vi "Leader8.vi"   [LabVIEW 2016]
uses:
  <vilib>/NXT/Block Support/NXT_TimerIndex.ctl
  <vilib>/NXT/Block Support/NXT_OutputPort.ctl
  <vilib>/NXT/Block Support/NXT_InputPort.ctl
  <vilib>/NXT/Dual Mode Library/Motors/ResetMotor.vi
  <vilib>/NXT/Dual Mode Library/Sensors/Reset_Timer.vi
  <vilib>/NXT/Dual Mode Library/Sensors/EV3_Color_Reflect.vi
  <vilib>/NXT/Dual Mode Library/Sensors/EV3_Gyro_Angle.vi
  <vilib>/NXT/Dual Mode Library/Sensors/Touch_Pressed.vi
  <vilib>/NXT/Dual Mode Library/Display/drawText.vi
  <vilib>/NXT/Dual Mode Library/Sensors/Read_Timer.vi
  <vilib>/NXT/Dual Mode Library/Display/drawNumber.vi
  <vilib>/NXT/Dual Mode Library/Motors/Rotation.vi
  <vilib>/NXT/Dual Mode Library/Sensors/EV3_Gyro_Reset.vi
  <vilib>/NXT/Dual Mode Library/Sensors/EV3_Gyro_Rate.vi
  <vilib>/NXT/Dual Mode Library/Display/drawNumber_float.vi
  <vilib>/NXT/Dual Mode Library/prims/inRangeAndCoerce/inRangeAndCoerce_float.vi
  <vilib>/NXT/NXTIO Xnodes/NXTIONodeSubVIs/NXTMoveMotors.vi
  <vilib>/NXT/Dual Mode Library/Display/drawText_Right.vi
  <vilib>/NXT/NXTIO Xnodes/NXTIONodeSubVIs/NXTStopMotors.vi
  <vilib>/NXT/Subs/LVHSConnector.ctl
  <vilib>/NXT/NXTIO Xnodes/AddressXNode/NXTIOAddress.xnode
  <vilib>/NXT/NXTIO Xnodes/NXTIOXNode/NXTIO.xnode
  <vilib>/NXT/LegoClasses/BrickReference/BrickReference.lvclass
types:
  T1 = typedef "LVHSConnector.ctl" = refnum<class "BrickReference.lvclass">
  T2 = typedef "NXT_InputPort.ctl" = u32
  T3 = typedef "NXT_OutputPort.ctl" = u8
  T4 = typedef "NXT_TimerIndex.ctl" = u8
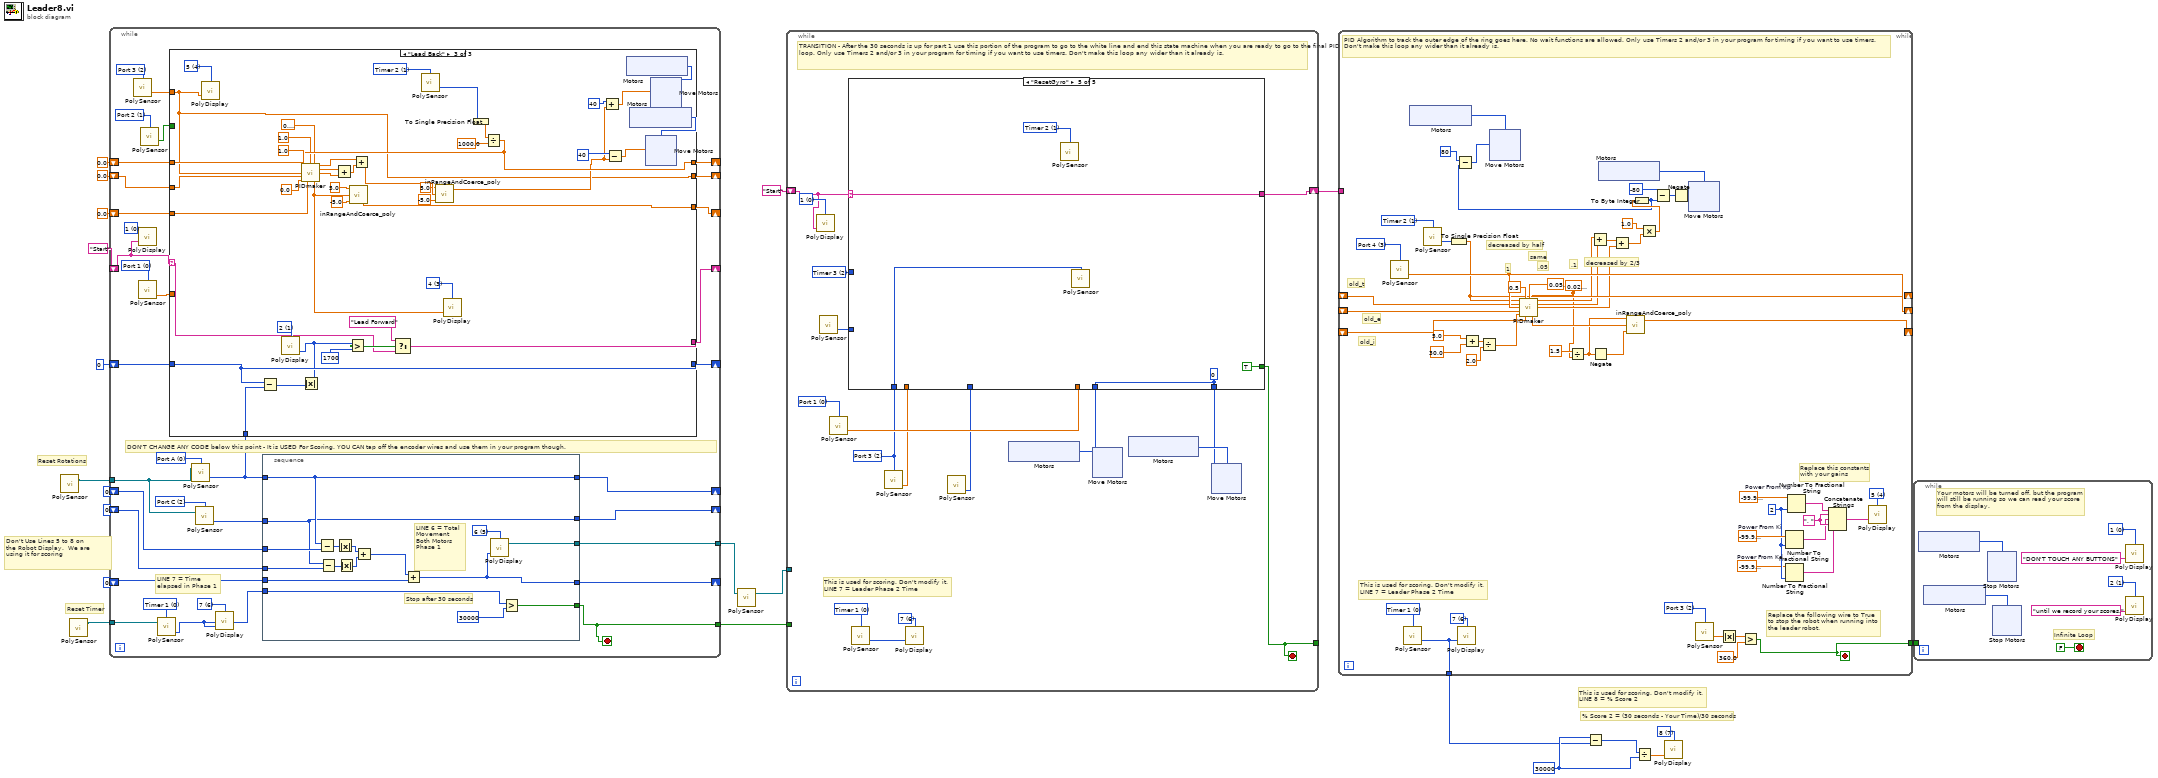
[diagram p0: block diagram]
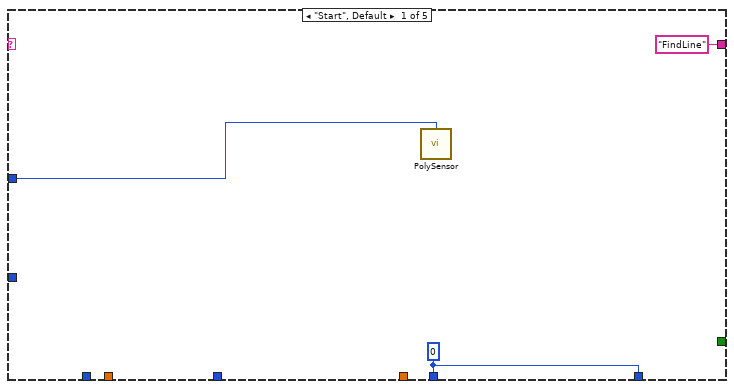
[diagram p2: hidden frame]
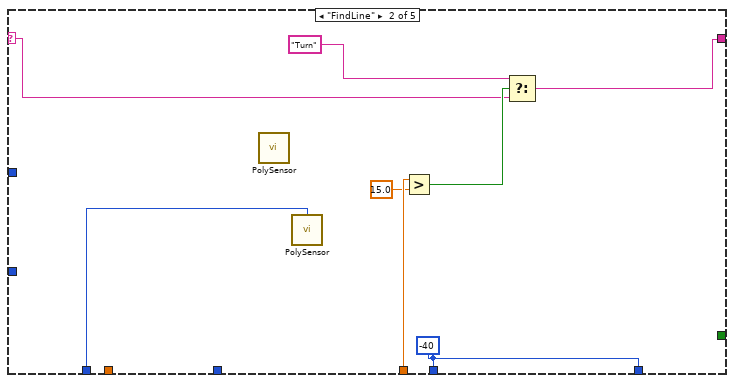
[diagram p3: hidden frame]
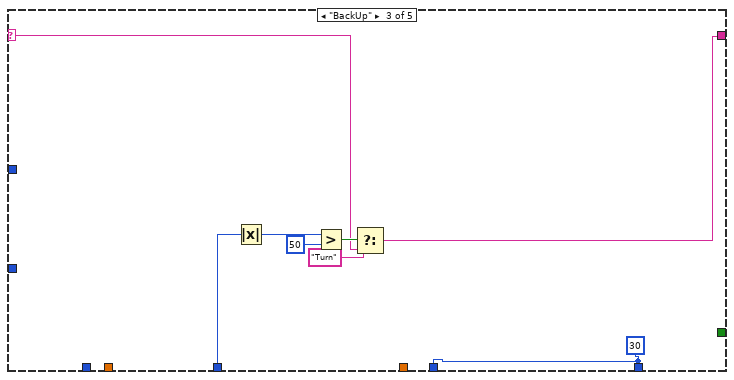
[diagram p4: hidden frame]
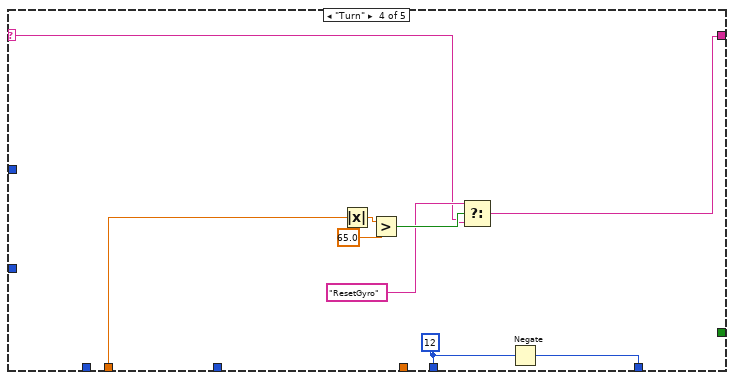
[diagram p5: hidden frame]
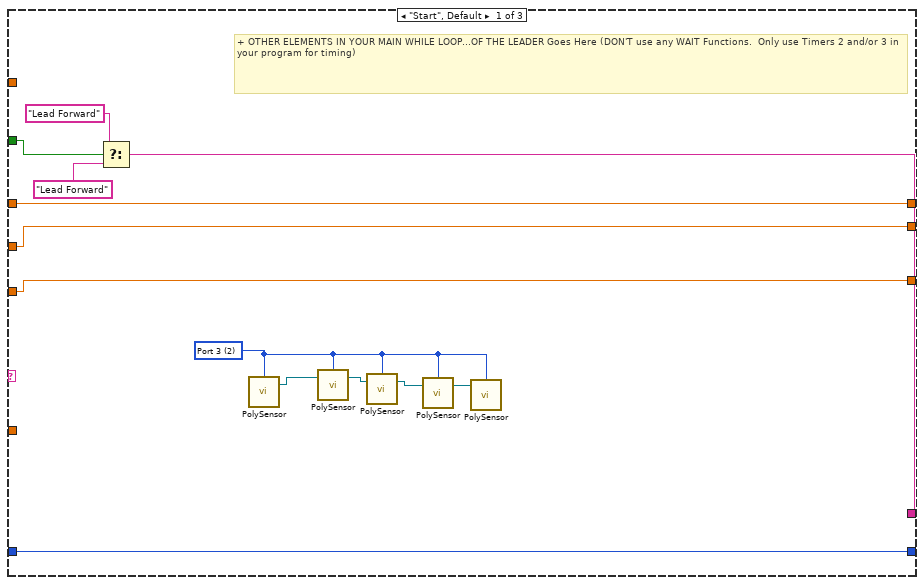
[diagram p6: hidden frame]
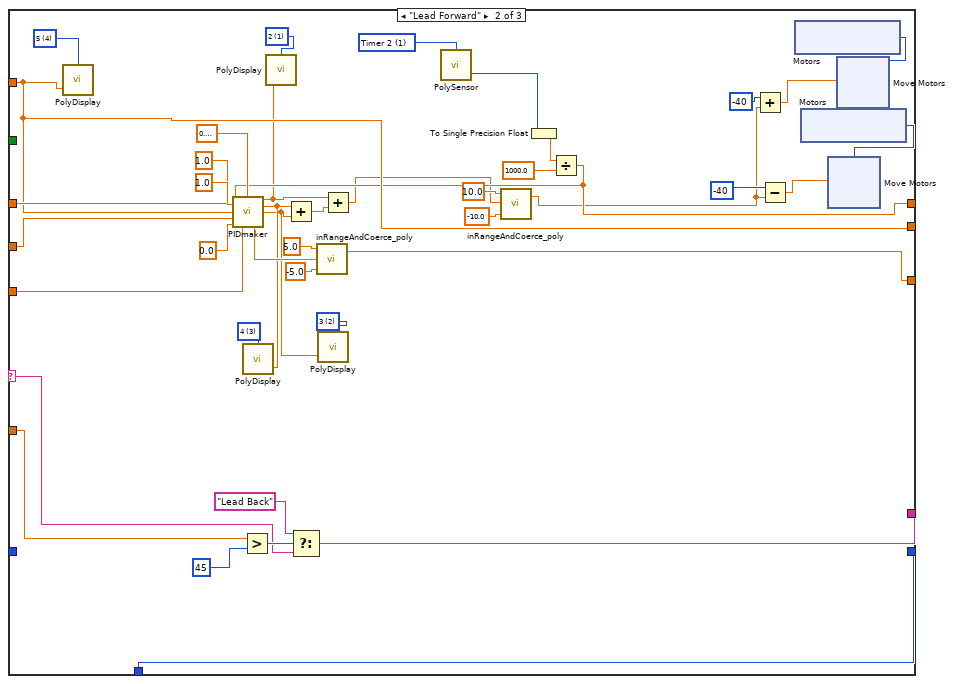
[diagram p7: hidden frame]
diagram:
  w6 = u32 30000 ("Value (msec)")
  w7 = i16 7 items=["1", "2", "3", "4", "5", "6", "7", "8", "9", "10", "11", "12"] ("Line")
  # "This is used for scoring. Don't modify it.\nLINE 8 = % Score 2"
  # "% Score 2 = (30 seconds - Your Time)/30 seconds"
  # "Don't Use Lines 5 to 8 on\nthe Robot Display.  We are \nusing it for scoring"
  # "Reset Timer"
  # "Reset Rotations"
  n1 = call-poly <vilib>:"PolySensor.vi"() -> ("NXT/EV3"=w18:T1)  [unwired: 4 in]
  n2 = call-poly <vilib>:"PolySensor.vi"() -> ("NXT/EV3"=w17:T1)  [unwired: 4 in]
  n3 = while {
    tunnel: w18 -> [w55]
    shift-right: [w50] -> _
    shift-left: 0 ("Angle of Rotation") -> [w52]
    shift-right: [w49] -> _
    shift-left: 0 ("Angle of Rotation") -> [w51]
    shift-right: [w53] -> _
    shift-left: 0 -> [w54]
    tunnel: w17 -> [w47]
    tunnel: [w24] -> w1
    tunnel: [w42] -> w16
    shift-right: [w36] -> _
    shift-left: 0 -> [w37]
    shift-right: [w32] -> _
    shift-left: "Start" -> [w31]
    shift-right: [w26] -> _
    shift-left: sgl 0.0 -> [w29]
    shift-right: [w25] -> _
    shift-left: sgl 0.0 ("Degrees") -> [w30]
    shift-right: [w27] -> _
    shift-left: sgl 0.0 ("coerced(x)") -> [w28]
    stop <- w24 stop-if-true
    w23 = T2 1 items=["Port 1", "Port 2", "Port 3", "Port 4"] ("Port (Port 1)")
    w33 = i16 0 items=["1", "2", "3", "4", "5", "6", "7", "8", "9", "10", "11", "12"] ("Line")
    w35 = T2 2 items=["Port 1", "Port 2", "Port 3", "Port 4"] ("Port (Port 1)")
    w38 = T2 0 items=["Port 1", "Port 2", "Port 3", "Port 4"] ("Port (Port 1)")
    w44 = i16 6 items=["1", "2", "3", "4", "5", "6", "7", "8", "9", "10", "11", "12"] ("Line")
    w45 = T3 0 items=["Port A", "Port B", "Port C", "Port D"] ("Port (Port A)")
    w46 = T3 2 items=["Port A", "Port B", "Port C", "Port D"] ("Port (Port A)")
    w48 = T4 0 items=["Timer 1", "Timer 2", "Timer 3"] ("Timer (Timer 1)")
    # "DON'T CHANGE ANY CODE below this point - It is USED For Scoring. YOU CAN tap off the encoder wires and use them in your program though."
    # "LINE 7 = Time elapsed in Phase 1"
    n4 = call-poly <vilib>:"PolySensor.vi"("Port (Port 1)"=w35) -> ("Degrees"=w34:sgl)  [unwired: 2 in, 1 out]
    n5 = call-poly <vilib>:"PolyDisplay.vi"("Text"=w31, "Line"=w33) -> ()  [unwired: 2 in, 1 out]
    n6 = call-poly <vilib>:"PolySensor.vi"("Port (Port 1)"=w38) -> ("Scaled Value"=w22:sgl)  [unwired: 2 in, 1 out]
    n7 = call-poly <vilib>:"PolySensor.vi"("Port (Port 1)"=w23) -> ("Yes / No"=w41:bool)  [unwired: 2 in, 1 out]
    n8 = call-poly <vilib>:"PolySensor.vi"("NXT/EV3"=w47, "Timer (Timer 1)"=w48) -> ("Value (msec)"=w43:u32)  [unwired: 1 in, 1 out]
    n9 = call-poly <vilib>:"PolySensor.vi"("NXT/EV3"=w55, "Port (Port A)"=w45) -> ("Angle of Rotation"=w40:i32)  [unwired: 1 in, 1 out]
    n10 = case shown="\"Lead Back\"" w31 {
      selector: w31 -> [_ w106 w160]
      tunnel: [w67 w107 w164] -> w32
      tunnel: w41 -> [w68 _ _]
      tunnel: w40 -> [_ w104 w161]
      tunnel: w37 -> [w65 _ w159]
      tunnel: w22 -> [_ w105 _]
      tunnel: [w65 w104 w159] -> w36
      tunnel: w34 -> [_ w81 w127]
      tunnel: w30 -> [w63 w86 w145]
      tunnel: w29 -> [w64 w87 w144]
      tunnel: w28 -> [w62 w85 w139]
      tunnel: [w62 w84 w138] -> w27
      tunnel: [w64 w80 w135] -> w26
      tunnel: [w63 w81 w127] -> w25
      frame "Start", Default {
        w57 = T2 2 items=["Port 1", "Port 2", "Port 3", "Port 4"] ("Port (Port 1)")
        # "+ OTHER ELEMENTS IN YOUR MAIN WHILE LOOP...OF THE LEADER Goes Here (DON'T use any WAIT Functions.  Only use Timers 2 and/or 3 in your program for timing)"
        n11 = Select(t="Lead Forward", s=w68, f="Lead Forward") -> (s? t:f=w67:string)
        n12 = call-poly <vilib>:"PolySensor.vi"("Port (Port 1)"=w57) -> ("NXT/EV3"=w58:T1)  [unwired: 3 in]
        n13 = call-poly <vilib>:"PolySensor.vi"("NXT/EV3"=w58, "Port (Port 1)"=w57) -> ("NXT/EV3"=w59:T1)  [unwired: 1 in, 1 out]
        n14 = call-poly <vilib>:"PolySensor.vi"("NXT/EV3"=w59, "Port (Port 1)"=w57) -> ("NXT/EV3"=w61:T1)  [unwired: 1 in, 1 out]
        n15 = call-poly <vilib>:"PolySensor.vi"("NXT/EV3"=w61, "Port (Port 1)"=w57) -> ("NXT/EV3"=w60:T1)  [unwired: 1 in, 1 out]
        n16 = call-poly <vilib>:"PolySensor.vi"("NXT/EV3"=w60, "Port (Port 1)"=w57) -> ()  [unwired: 2 in, 1 out]
      }
      frame "Lead Forward" {
        w70 = i16 2 items=["1", "2", "3", "4", "5", "6", "7", "8", "9", "10", "11", "12"] ("Line")
        w72 = i16 1 items=["1", "2", "3", "4", "5", "6", "7", "8", "9", "10", "11", "12"] ("Line")
        w75 = i16 3 items=["1", "2", "3", "4", "5", "6", "7", "8", "9", "10", "11", "12"] ("Line")
        w82 = i16 4 items=["1", "2", "3", "4", "5", "6", "7", "8", "9", "10", "11", "12"] ("Line")
        w92 = T4 1 items=["Timer 1", "Timer 2", "Timer 3"] ("Timer (Timer 1)")
        n17 = call-poly <vilib>:"PolyDisplay.vi"("number"=w81, "Line"=w82) -> ()  [unwired: 2 in, 1 out]
        n18 = Greater?(x=w105, y=45) -> (0:w108:bool)
        n19 = Select(t="Lead Back", s=w108, f=w106) -> (s? t:f=w107:string)
        n20 = call-poly <vilib>:"PolySensor.vi"("Timer (Timer 1)"=w92) -> ("Value (msec)"=w91:u32)  [unwired: 2 in, 1 out]
        n21 = To Single Precision Float(number=w91) -> (single precision float=w89:sgl)
        n22 = Divide(x=w89, y=sgl 1000.0) -> (x/y=w80:sgl)
        n23 = call "PIDmaker.vi"("New Time"=w80, "Kp"=sgl 1.0, "Kd"=sgl 1.0, "Ki"=sgl 0.1, "Old Time"=w87, "New Value"=w81, "Old Value"=w86, "Desired Value"=sgl 0.0, "Integral In"=w85) -> ("P out"=w73:sgl, "D out"=w71:sgl, "I out"=w69:sgl, "Integral Out"=w74:sgl)  [unwired: 3 in]
        n24 = call-poly <vilib>:"PolyDisplay.vi"("number"=w71, "Line"=w75) -> ()  [unwired: 2 in, 1 out]
        n25 = call-poly <vilib>:"PolyDisplay.vi"("number"=w73, "Line"=w72) -> ()  [unwired: 2 in, 1 out]
        n26 = Add(x=w71, y=w69) -> (x+y=w100:sgl)
        n27 = call-poly <vilib>:"inRangeAndCoerce_poly.vi"("lower limit"=sgl -5.0, "x"=w74, "upper limit"=sgl 5.0) -> ("coerced(x)"=w84:sgl)  [unwired: 1 out]
        n28 = call-poly <vilib>:"PolyDisplay.vi"("number"=w69, "Line"=w70) -> ()  [unwired: 2 in, 1 out]
        n29 = Add(x=w73, y=w100) -> (x+y=w77:sgl)
        n30 = call-poly <vilib>:"inRangeAndCoerce_poly.vi"("lower limit"=sgl -10.0, "x"=w77, "upper limit"=sgl 10.0) -> ("coerced(x)"=w76:sgl)  [unwired: 1 out]
        n31 = Add(x=-40, y=w76) -> (x+y=w93:sgl)
        n32 = Subtract(x=-40, y=w76) -> (x-y=w83:sgl)
        n33 = xnode "Motors"() -> ("Motor"=w103:T3)
        n34 = xnode "Motors"() -> ("Motor"=w88:T3)
        n35 = xnode "Move Motors"("Power/Speed 1"=w83, "Motors"=w88) -> ()  [unwired: 1 in, 1 out]
        n36 = xnode "Move Motors"("Power/Speed 1"=w93, "Motors"=w103) -> ()  [unwired: 1 in, 1 out]
      }
      frame "Lead Back" {
        w128 = i16 4 items=["1", "2", "3", "4", "5", "6", "7", "8", "9", "10", "11", "12"] ("Line")
        w143 = T4 1 items=["Timer 1", "Timer 2", "Timer 3"] ("Timer (Timer 1)")
        w165 = i16 3 items=["1", "2", "3", "4", "5", "6", "7", "8", "9", "10", "11", "12"] ("Line")
        w168 = i16 1 items=["1", "2", "3", "4", "5", "6", "7", "8", "9", "10", "11", "12"] ("Line")
        n37 = call-poly <vilib>:"PolyDisplay.vi"("number"=w127, "Line"=w128) -> ()  [unwired: 2 in, 1 out]
        n38 = Subtract(x=w159, y=w161) -> (x-y=w158:i32)
        n39 = Absolute Value(x=w158) -> (abs(x)=w157:i32)
        n40 = call-poly <vilib>:"PolyDisplay.vi"("number"=w157, "Line"=w168) -> ()  [unwired: 2 in, 1 out]
        n41 = Greater?(x=w157, y=1700) -> (0:w162:bool)
        n42 = Select(t="Lead Forward", s=w162, f=w160) -> (s? t:f=w164:string)
        n43 = call-poly <vilib>:"PolySensor.vi"("Timer (Timer 1)"=w143) -> ("Value (msec)"=w142:u32)  [unwired: 2 in, 1 out]
        n44 = To Single Precision Float(number=w142) -> (single precision float=w140:sgl)
        n45 = Divide(x=w140, y=sgl 1000.0) -> (x/y=w135:sgl)
        n46 = call "PIDmaker.vi"("New Time"=w135, "Kp"=sgl 1.0, "Kd"=sgl 1.0, "Ki"=sgl 0.1, "Old Time"=w144, "New Value"=w127, "Old Value"=w145, "Desired Value"=sgl 0.0, "Integral In"=w139) -> ("P out"=w152:sgl, "D out"=w153:sgl, "I out"=w150:sgl, "Integral Out"=w137:sgl)  [unwired: 3 in]
        n47 = Add(x=w153, y=w150) -> (x+y=w154:sgl)
        n48 = call-poly <vilib>:"inRangeAndCoerce_poly.vi"("lower limit"=sgl -5.0, "x"=w137, "upper limit"=sgl 5.0) -> ("coerced(x)"=w138:sgl)  [unwired: 1 out]
        n49 = Add(x=w152, y=w154) -> (x+y=w132:sgl)
        n50 = call-poly <vilib>:"inRangeAndCoerce_poly.vi"("lower limit"=sgl -5.0, "x"=w132, "upper limit"=sgl 5.0) -> ("coerced(x)"=w131:sgl)  [unwired: 1 out]
        n51 = call-poly <vilib>:"PolyDisplay.vi"("number"=w137, "Line"=w165) -> ()  [unwired: 2 in, 1 out]
        n52 = Add(x=40, y=w131) -> (x+y=w146:sgl)
        n53 = Subtract(x=40, y=w131) -> (x-y=w136:sgl)
        n54 = xnode "Motors"() -> ("Motor"=w166:T3)
        n55 = xnode "Motors"() -> ("Motor"=w167:T3)
        n56 = xnode "Move Motors"("Power/Speed 1"=w136, "Motors"=w167) -> ()  [unwired: 1 in, 1 out]
        n57 = xnode "Move Motors"("Power/Speed 1"=w146, "Motors"=w166) -> ()  [unwired: 1 in, 1 out]
      }
    }
    n58 = call-poly <vilib>:"PolySensor.vi"("NXT/EV3"=w55, "Port (Port A)"=w46) -> ("Angle of Rotation"=w39:i32)  [unwired: 1 in, 1 out]
    n59 = call-poly <vilib>:"PolyDisplay.vi"("number"=w43, "Line"=w44) -> ()  [unwired: 2 in, 1 out]
    n60 = stacked-sequence {
      tunnel: w54 -> [w201]
      tunnel: [w188] -> w53
      tunnel: w43 -> [w199]
      tunnel: [w198] -> w24
      tunnel: w40 -> [w191]
      tunnel: w39 -> [w190]
      tunnel: w52 -> [w193]
      tunnel: w51 -> [w192]
      tunnel: [w191] -> w50
      tunnel: [w190] -> w49
      tunnel: [w186] -> w42
      frame #0 {
        w187 = i16 5 items=["1", "2", "3", "4", "5", "6", "7", "8", "9", "10", "11", "12"] ("Line")
        # "LINE 6 = Total\nMovement\nBoth Motors\nPhase 1"
        # "Stop after 30 seconds"
        n61 = Subtract(x=w191, y=w193) -> (x-y=w197:i32)
        n62 = Subtract(x=w190, y=w192) -> (x-y=w196:i32)
        n63 = Absolute Value(x=w197) -> (abs(x)=w195:i32)
        n64 = Absolute Value(x=w196) -> (abs(x)=w194:i32)
        n65 = Add(x=w195, y=w194) -> (x+y=w189:i32)
        n66 = Add(x=w189, y=w201) -> (x+y=w188:i32)
        n67 = call-poly <vilib>:"PolyDisplay.vi"("number"=w188, "Line"=w187) -> ("NXT/EV3"=w186:T1)  [unwired: 2 in]
        n68 = Greater?(x=w199, y=u32 30000 ("Value (msec)")) -> (0:w198:bool)
      }
    }
  }
  n69 = call-poly <vilib>:"PolySensor.vi"("NXT/EV3"=w16) -> ("NXT/EV3"=w2:T1)  [unwired: 3 in]
  n70 = while {
    shift-right: [w206] -> w8
    shift-left: "Start" -> [w202]
    tunnel: [w204] -> _
    tunnel: w2 -> [_]
    tunnel: w1 -> [_]
    stop <- w204 stop-if-true
    w203 = i16 0 items=["1", "2", "3", "4", "5", "6", "7", "8", "9", "10", "11", "12"] ("Line")
    w205 = T2 0 items=["Port 1", "Port 2", "Port 3", "Port 4"] ("Port (Port 1)")
    w209 = T2 2 items=["Port 1", "Port 2", "Port 3", "Port 4"] ("Port (Port 1)")
    w214 = T4 2 items=["Timer 1", "Timer 2", "Timer 3"] ("Timer (Timer 1)")
    w217 = i16 6 items=["1", "2", "3", "4", "5", "6", "7", "8", "9", "10", "11", "12"] ("Line")
    w219 = T4 0 items=["Timer 1", "Timer 2", "Timer 3"] ("Timer (Timer 1)")
    # "This is used for scoring. Don't modify it.\nLINE 7 = Leader Phase 2 Time"
    # "TRANSITION - After the 30 seconds is up for part 1 use this portion of the program to go to the white line and end this state machine when you are ready to go to the final PID control loop. Only use Timers 2 and/or 3 in your program for timing if you want to use timers. Don't make this loop any wider than it already is."
    n71 = call-poly <vilib>:"PolyDisplay.vi"("Text"=w202, "Line"=w203) -> ()  [unwired: 2 in, 1 out]
    n72 = call-poly <vilib>:"PolySensor.vi"() -> ("Value (msec)"=w213:u32)  [unwired: 3 in, 1 out]
    n73 = call-poly <vilib>:"PolySensor.vi"("Port (Port 1)"=w205) -> ("Scaled Value"=w210:sgl)  [unwired: 2 in, 1 out]
    n74 = call-poly <vilib>:"PolySensor.vi"("Timer (Timer 1)"=w219) -> ("Value (msec)"=w218:u32)  [unwired: 2 in, 1 out]
    n75 = call-poly <vilib>:"PolySensor.vi"("Port (Port 1)"=w209) -> ("Degrees"=w208:sgl)  [unwired: 2 in, 1 out]
    n76 = call-poly <vilib>:"PolyDisplay.vi"("number"=w218, "Line"=w217) -> ()  [unwired: 2 in, 1 out]
    n77 = call-poly <vilib>:"PolySensor.vi"() -> ("Angle of Rotation"=w207:i32)  [unwired: 3 in, 1 out]
    n78 = case shown="\"ResetGyro\"" w202 {
      selector: w202 -> [_ w241 w249 w256 w266]
      tunnel: ["FindLine" w243 w247 w255 w266] -> w206
      tunnel: w214 -> [w238 _ _ _ _]
      tunnel: w213 -> [_ _ _ _ _]
      tunnel: [w236 w239 w254 w263 w265] -> w212
      tunnel: [w236 w239 w254 w262 w265] -> w211
      tunnel: w210 -> [_ w246 _ _ _]
      tunnel: w209 -> [_ w240 _ _ w268]
      tunnel: w208 -> [_ _ _ w261 _]
      tunnel: w207 -> [_ _ w253 _ _]
      tunnel: [_ _ _ _ TRUE] -> w204
      frame "Start", Default {
        w236 = 0
        n79 = call-poly <vilib>:"PolySensor.vi"("Timer (Timer 1)"=w238) -> ()  [unwired: 3 in, 1 out]
      }
      frame "FindLine" {
        w239 = -40
        n80 = call-poly <vilib>:"PolySensor.vi"() -> ()  [unwired: 4 in, 1 out]
        n81 = call-poly <vilib>:"PolySensor.vi"("Port (Port 1)"=w240) -> ()  [unwired: 3 in, 1 out]
        n82 = Greater?(x=w246, y=sgl 15.0) -> (0:w244:bool)
        n83 = Select(t="Turn", s=w244, f=w241) -> (s? t:f=w243:string)
      }
      frame "BackUp" {
        w254 = 30
        n84 = Absolute Value(x=w253) -> (abs(x)=w251:i32)
        n85 = Greater?(x=w251, y=50) -> (0:w250:bool)
        n86 = Select(t="Turn", s=w250, f=w249) -> (s? t:f=w247:string)
      }
      frame "Turn" {
        w263 = 12
        n87 = Absolute Value(x=w261) -> (abs(x)=w260:sgl)
        n88 = Greater?(x=w260, y=sgl 65.0) -> (0:w258:bool)
        n89 = Select(t="ResetGyro", s=w258, f=w256) -> (s? t:f=w255:string)
        n90 = Negate(x=w263) -> (-x=w262:i32)
      }
      frame "ResetGyro" {
        w264 = T4 1 items=["Timer 1", "Timer 2", "Timer 3"] ("Timer (Timer 1)")
        w265 = 0
        n91 = call-poly <vilib>:"PolySensor.vi"("Timer (Timer 1)"=w264) -> ()  [unwired: 3 in, 1 out]
        n92 = call-poly <vilib>:"PolySensor.vi"("Port (Port 1)"=w268) -> ()  [unwired: 3 in, 1 out]
      }
    }
    n93 = xnode "Motors"() -> ("Motor"=w216:T3)
    n94 = xnode "Move Motors"("Power/Speed 1"=w212, "Motors"=w216) -> ()  [unwired: 1 in, 1 out]
    n95 = xnode "Motors"() -> ("Motor"=w215:T3)
    n96 = xnode "Move Motors"("Power/Speed 1"=w211, "Motors"=w215) -> ()  [unwired: 1 in, 1 out]
  }
  n97 = while {
    tunnel: [w273] -> w9
    tunnel: w8 -> [_]
    tunnel: [w320] -> w5
    shift-right: [w305] -> _
    shift-left: _ -> [w304]
    shift-right: [w301] -> _
    shift-left: _ -> [w300]
    shift-right: [w288] -> _
    shift-left: _ -> [w289]
    stop <- w273 stop-if-true
    w277 = T2 2 items=["Port 1", "Port 2", "Port 3", "Port 4"] ("Port (Port 1)")
    w286 = sgl 0.03 ("Ki")
    w307 = T4 1 items=["Timer 1", "Timer 2", "Timer 3"] ("Timer (Timer 1)")
    w308 = T2 3 items=["Port 1", "Port 2", "Port 3", "Port 4"] ("Port (Port 1)")
    w313 = ", " ("string")
    w316 = i16 2 ("precision (6)")
    w315 = sgl -99.9  # Power From Kd
    w317 = sgl -99.9  # Power From Ki
    w318 = sgl -99.9  # Power From Kp
    w319 = i16 4 items=["1", "2", "3", "4", "5", "6", "7", "8", "9", "10", "11", "12"] ("Line")
    w321 = i16 6 items=["1", "2", "3", "4", "5", "6", "7", "8", "9", "10", "11", "12"] ("Line")
    w322 = T4 0 items=["Timer 1", "Timer 2", "Timer 3"] ("Timer (Timer 1)")
    # "decreased by 2/3"
    # "same"
    # "decreased by half"
    # ".1"
    # ".05"
    # "1"
    # "old_i"
    # "old_e"
    # "old_t"
    # "Replace this constants\nwith your gains"
    # "This is used for scoring. Don't modify it.\nLINE 7 = Leader Phase 2 Time"
    # "PID Algorithm to track the outer edge of the ring goes here. No wait functions are allowed. Only use Timers 2 and/or 3 in your program for timing if you want to use timers.\nDon't make this loop any wider than it already is."
    # "Replace the following wire to True\nto stop the robot when running into \nthe leader robot."
    n98 = call-poly <vilib>:"PolySensor.vi"("Port (Port 1)"=w308) -> ("Scaled Value"=w305:sgl)  [unwired: 2 in, 1 out]
    n99 = call-poly <vilib>:"PolySensor.vi"("Timer (Timer 1)"=w322) -> ("Value (msec)"=w320:u32)  [unwired: 2 in, 1 out]
    n100 = xnode "Motors"() -> ("Motor"=w283:T3)
    n101 = call-poly <vilib>:"PolySensor.vi"("Timer (Timer 1)"=w307) -> ("Value (msec)"=w306:u32)  [unwired: 2 in, 1 out]
    n102 = To Single Precision Float(number=w306) -> (single precision float=w301:sgl)
    n103 = call-poly <vilib>:"PolyDisplay.vi"("number"=w320, "Line"=w321) -> ()  [unwired: 2 in, 1 out]
    n104 = Add(x=sgl 5.0, y=sgl 30.0) -> (x+y=w299:sgl)
    n105 = Divide(x=w299, y=sgl 2.0) -> (x/y=w296:sgl)
    n106 = call "PIDmaker.vi"("New Time"=w301, "Kp"=sgl 0.5, "Kd"=sgl 0.05, "Ki"=w286, "Old Time"=w300, "New Value"=w305, "Old Value"=w304, "Desired Value"=w296, "Integral In"=w289) -> ("P out"=w292:sgl, "D out"=w291:sgl, "I out"=w290:sgl, "Integral Out"=w295:sgl)  [unwired: 3 in]
    n107 = Divide(x=sgl 1.5, y=w286) -> (x/y=w284:sgl)
    n108 = Add(x=w292, y=w291) -> (x+y=w293:sgl)
    n109 = Negate(x=w284) -> (-x=w285:sgl)
    n110 = xnode "Motors"() -> ("Motor"=w309:T3)
    n111 = Add(x=w293, y=w290) -> (x+y=w279:sgl)
    n112 = call-poly <vilib>:"inRangeAndCoerce_poly.vi"("lower limit"=w285, "x"=w295, "upper limit"=w284) -> ("coerced(x)"=w288:sgl)  [unwired: 1 out]
    n113 = Multiply(x=sgl 1.0 ("Ki"), y=w279) -> (x*y=w271:sgl)
    n114 = To Byte Integer(number=w271) -> (8bit integer=w269:i8)
    n115 = Subtract(x=i8 80 ("Power/Speed 1"), y=w269) -> (x-y=w270:i8)
    n116 = xnode "Move Motors"("Power/Speed 1"=w270, "Motors"=w283) -> ()  [unwired: 1 in, 1 out]
    n117 = Subtract(x=i8 -80, y=w269) -> (x-y=w281:i8)
    n118 = Negate(x=w281) -> (-x=w280:i8)
    n119 = xnode "Move Motors"("Power/Speed 1"=w280, "Motors"=w309) -> ()  [unwired: 1 in, 1 out]
    n120 = call-poly <vilib>:"PolySensor.vi"("Port (Port 1)"=w277) -> ("Degrees"=w276:sgl)  [unwired: 2 in, 1 out]
    n121 = Absolute Value(x=w276) -> (abs(x)=w274:sgl)
    n122 = Greater?(x=w274, y=sgl 360.0) -> (0:w273:bool)
    n123 = Number To Fractional String(number=w317, precision (6)=w316) -> (F-format string=w312:string)  [unwired: 2 in]
    n124 = Number To Fractional String(number=w315, precision (6)=w316) -> (F-format string=w311:string)  [unwired: 2 in]
    n125 = Number To Fractional String(number=w318, precision (6)=w316) -> (F-format string=w314:string)  [unwired: 2 in]
    n126 = Concatenate Strings(w314, w313, w312, w313, w311) -> (w310:string)
    n127 = call-poly <vilib>:"PolyDisplay.vi"("Text"=w310, "Line"=w319) -> ()  [unwired: 2 in, 1 out]
  }
  n128 = Subtract(x=w6, y=w5) -> (x-y=w4:u32)
  n129 = Divide(x=w4, y=w6) -> (x/y=w3:dbl)
  n130 = call-poly <vilib>:"PolyDisplay.vi"("number"=w3, "Line"=w7) -> ()  [unwired: 2 in, 1 out]
  n131 = while {
    tunnel: w9 -> [_]
    stop <- FALSE stop-if-true
    w339 = i16 1 items=["1", "2", "3", "4", "5", "6", "7", "8", "9", "10", "11", "12"] ("Line")
    w342 = i16 0 items=["1", "2", "3", "4", "5", "6", "7", "8", "9", "10", "11", "12"] ("Line")
    # "Your motors will be turned off, but the program\nwill still be running so we can read your score\nfrom the display."
    # "Infinite Loop"
    n132 = xnode "Motors"() -> ("Motor"=w344:T3)
    n133 = xnode "Motors"() -> ("Motor"=w343:T3)
    n134 = xnode "Stop Motors"("Motors"=w344) -> ()  [unwired: 1 in, 1 out]
    n135 = xnode "Stop Motors"("Motors"=w343) -> ()  [unwired: 1 in, 1 out]
    n136 = call-poly <vilib>:"PolyDisplay.vi"("Text"="DON'T TOUCH ANY BUTTONS", "Line"=w342) -> ()  [unwired: 2 in, 1 out]
    n137 = call-poly <vilib>:"PolyDisplay.vi"("Text"="until we record your scores.", "Line"=w339) -> ()  [unwired: 2 in, 1 out]
  }
